vi "AndorConvertErrCodeToMessage.vi"(8 "function return":u32, 11 "Array":cluster{i32, string}[](array[cluster])) -> (0 "Element Return":cluster{i32, string}, 3 "Array out":cluster{i32, string}[](array[cluster]))   [LabVIEW 2018]
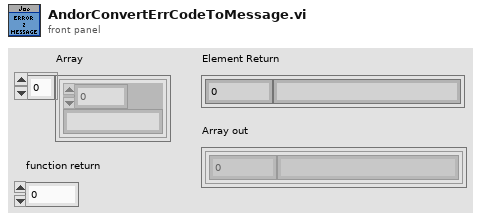
[diagram p1: front panel]
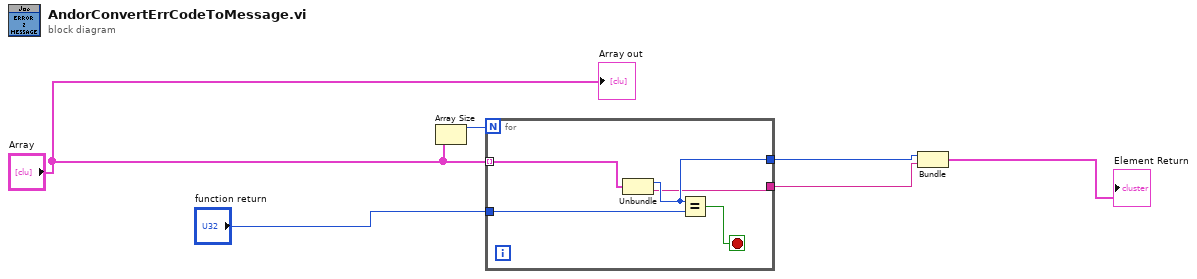
[diagram p0: block diagram]
diagram:
  n1 = Array Size(array="Array") -> (size(s)=w5:i32)
  n2 = for {
    N: w5 -> [_]
    tunnel: "Array" -> [w11] mode=indexing
    tunnel: "function return" -> [w10]
    tunnel: [w8] -> w3
    tunnel: [w7] -> w2
    stop <- w9 stop-if-true
    n3 = Unbundle(w11) -> (w8:i32, w7:string)
    n4 = Equal?(x=w8, y=w10) -> (x = y?=w9:bool)
  }
  n5 = Bundle(w3, w2) -> (→"Element Return":cluster{i32, string})  [unwired: 1 in]
  "Array out" <- "Array"
